vi "SplitConnectionTypeAndName.vi"(0 "Name + connectionType":string) -> (1 "Connection Type":T1, 2 "Name":string)   [LabVIEW 2010]
uses:
  <vilib>/NXT/NXT Controls/ConnectionType.ctl
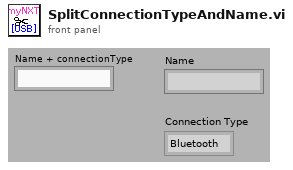
[diagram p1: front panel]
types:
  T1 = typedef "ConnectionType.ctl" = enum16{"Bluetooth", "USB"}
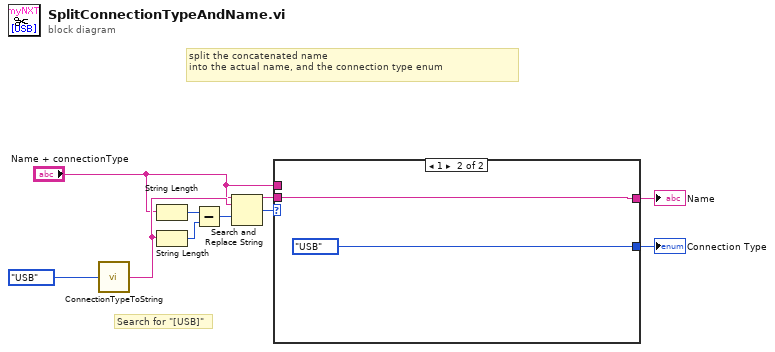
[diagram p0: block diagram]
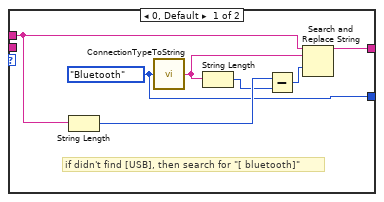
[diagram p2: hidden frame]
diagram:
  # "split the concatenated name\ninto the actual name, and the connection type enum"
  # "Search for \"[USB]\""
  n1 = call "ConnectionTypeToString.vi"("Connection Type"=ConnectionType."USB") -> ("String"=w10:string)
  n2 = String Length(string="Name + connectionType") -> (length=w1:i32)
  n3 = String Length(string=w10) -> (length=w4:i32)
  n4 = Subtract(x=w1, y=w4) -> (x-y=w2:i32)
  n5 = Search and Replace String(input string="Name + connectionType", search string=w10, offset=w2) -> (result string=w6:string, number of replacements=w3:i32)  [unwired: 5 in, 2 out]
  n6 = case shown="1" w3 {
    tunnel: "Name + connectionType" -> [w16 _]
    tunnel: w6 -> [_ w19]
    tunnel: [w17 w19] -> w7
    tunnel: [w12 ConnectionType."USB" ("Connection Type")] -> w8
    frame 0, Default {
      w12 = ConnectionType."Bluetooth" ("Connection Type")
      # "if didn't find [USB], then search for \"[ bluetooth]\""
      n7 = String Length(string=w16) -> (length=w15:i32)
      n8 = call "ConnectionTypeToString.vi"("Connection Type"=w12) -> ("String"=w11:string)
      n9 = String Length(string=w11) -> (length=w14:i32)
      n10 = Subtract(x=w15, y=w14) -> (x-y=w13:i32)
      n11 = Search and Replace String(input string=w16, search string=w11, offset=w13) -> (result string=w17:string)  [unwired: 5 in, 3 out]
    }
    frame 1 {
    }
  }
  "Connection Type" <- w8
  "Name" <- w7
